vi "RTS Macro Average Compressor Runtime.vi"(7 "Defrost/Cycle Times":dbl[](array[numeric]), 8 "Error In":errorcluster) -> (0 "Error Out":errorcluster, 1 "Average Compressor Power (Lower)":dbl, 2 "Filtered Compressor Run Time":dbl[](graph), 3 "Average Compressor Cycle Time (Min)":dbl)   [LabVIEW 2016]
uses:
  <vilib>/Analysis/baseanly.llb/Mean (DBL).vi
  <vilib>/gmath/statdist.llb/st_Percentiles (scalar).vi
  <vilib>/gmath/NI_Gmath.lvlib
  <vilib>/Analysis/NI_AALBase.lvlib
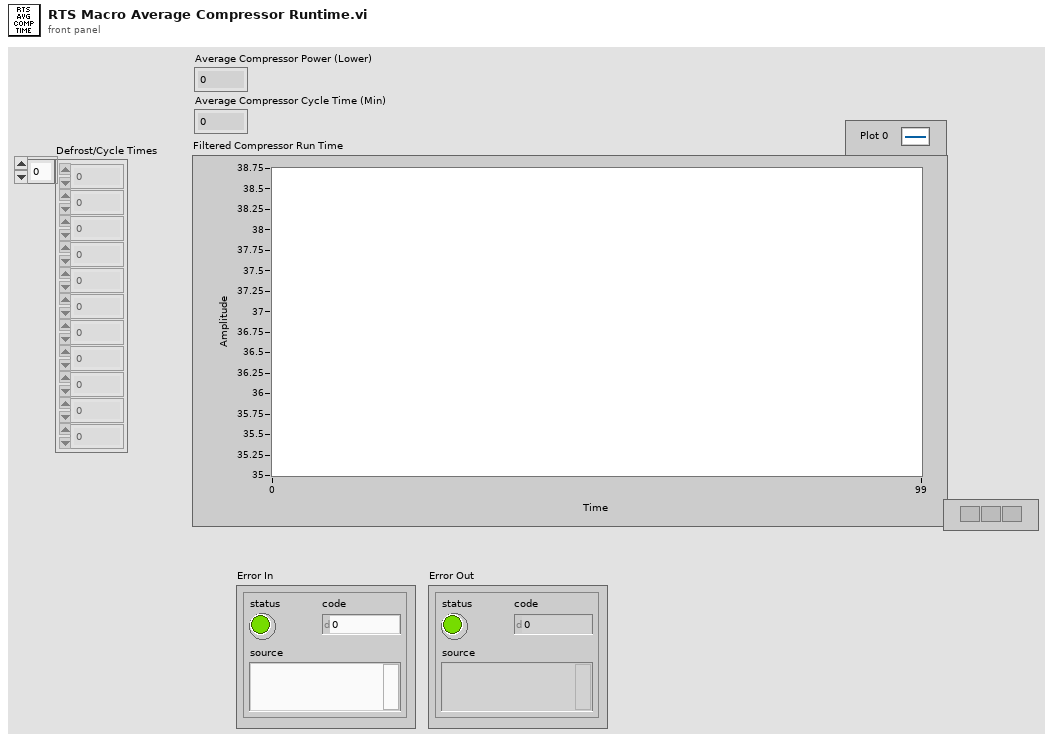
[diagram p1: front panel]
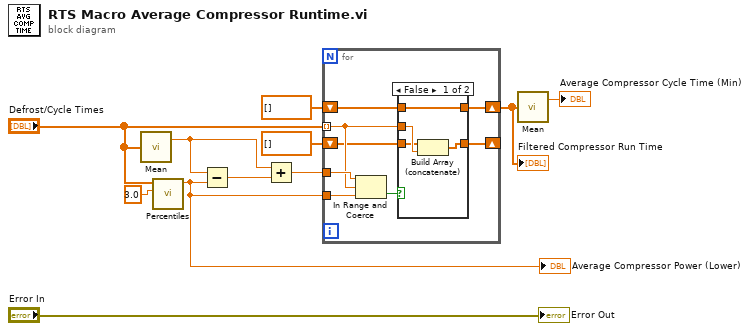
[diagram p0: block diagram]
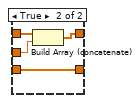
[diagram p2: hidden frame]
diagram:
  n1 = call-poly <vilib>:"Mean.vi"("X"="Defrost/Cycle Times") -> ("mean"=w6:dbl)  [unwired: 1 out]
  n2 = call-poly <vilib>:"Percentiles.vi"("p"=3.0, "x array"="Defrost/Cycle Times") -> ("percentile"=w5:dbl)  [unwired: 8 in, 1 out]
  "Average Compressor Power (Lower)" <- w5
  n3 = Subtract(x=w6, y=w5) -> (x-y=w3:dbl)
  n4 = Add(x=w6, y=w3) -> (x+y=w4:dbl)
  n5 = for {
    tunnel: w4 -> [w19]
    tunnel: w5 -> [w18]
    tunnel: "Defrost/Cycle Times" -> [w14] mode=indexing
    shift-right: [w15] -> w9
    shift-left: dbl[] [] -> [w16]
    shift-right: [w12] -> _
    shift-left: dbl[] [] -> [w13]
    n6 = In Range and Coerce(upper limit=w19, x=w14, lower limit=w18) -> (In Range?=w17:bool)  [unwired: 1 out]
    n7 = case shown="False" w17 {
      tunnel: w16 -> [w22 w27]
      tunnel: [w22 w26] -> w15
      tunnel: w14 -> [w23 w25]
      tunnel: w13 -> [w21 w24]
      tunnel: [w20 w24] -> w12
      frame False {
        n8 = Build Array (concatenate)(w21, w23) -> (w20:dbl[])
      }
      frame True {
        n9 = Build Array (concatenate)(w27, w25) -> (w26:dbl[])
      }
    }
  }
  "Filtered Compressor Run Time" <- w9
  n10 = call-poly <vilib>:"Mean.vi"("X"=w9) -> ("mean"=→"Average Compressor Cycle Time (Min)":dbl)  [unwired: 1 out]
  "Error Out" <- "Error In"
